vi "Set Win State.vi"(0 "reference in":refnum<class "GUI.lvclass">, 5 "WindowsState":T1, 11 "error in (no error)":errorcluster) -> (4 "reference out":refnum<class "GUI.lvclass">, 15 "error out":errorcluster)   [LabVIEW 2019, in "GUI.lvclass"]
uses:
  GUI.lvclass
  WindowsState.ctl
  GUI.lvclass/GUI.ctl
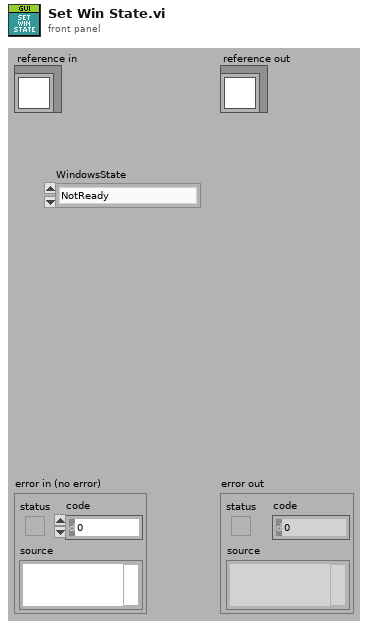
[diagram p1: front panel]
types:
  T1 = typedef "GUI.lvclass/WindowsState.ctl" = enum16{"NotReady", "Ready", "Inserted", "Opened"}
  T2 = typedef "GUI.lvclass/Shered Data.ctl" = cluster{"WindowsState":T1, "UI VI":refnum<vi>, "SubPnl":refnum<vi>}
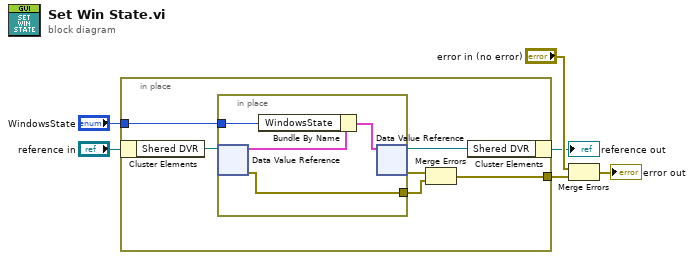
[diagram p0: block diagram]
diagram:
  n1 = in-place {
    in-place-border: [w8] -> w2
    in-place-border: "WindowsState" -> [w7]
    n2 = in-place-cluster #1("reference in") -> ("Shered DVR"=w12:refnum<data-value>)
    n3 = in-place {
      in-place-border: [w16] -> w9
      in-place-border: w7 -> [w13]
      n4 = in-place-dvr #2(w12) -> (w15:T2, w16:errorcluster)
      n5 = Bundle By Name(cluster=w15, "WindowsState"=w13) -> (w14:T2)
      n6 = in-place-dvr #2(w14) -> (w11:refnum<data-value>, w10:errorcluster)
    }
    n7 = Merge Errors(w10, w9) -> (w8:errorcluster)
    n8 = in-place-cluster #1("Shered DVR"=w11) -> (→"reference out":refnum<class "GUI.lvclass">)
  }
  n9 = Merge Errors("error in (no error)", w2) -> (→"error out":errorcluster)
